vi "Buffered Continuous Packets.vi"(0 "Input Buffer":string, 3 "Packet definitions":T2(array[cluster])=[{"Cmd/SOP Byte"="ª", "Header Size"=6, "Len"=5, "Chksum Start"=1, "Chksum End"=-4, "InHdr"=TRUE}, {"Cmd/SOP Byte"="Â", "Header Size"=1, "Len"=31, "Chksum Start"=0, "Chksum End"=-2, "InHdr"=FALSE}]) -> (4 "Number of Remainder Bytes":i32, 6 "Number of Valid Records Found":i32, 7 "Remainder String":string, 9 "Valid Records Found":string[](array[string]), 10 "# of Bytes Rejected":i32)   [LabVIEW 2017]
panel:
  out "SOP":bool=TRUE
  in  "Current Pkt Definition":T1
  out "length":i32
  # "This VI pulls packets from the incoming data stream and outputs them in an array.  The only packets recognized are those that match one of the entries in the packet definitions array.   The types of packets recognized are either the single byte Inertia-Link/GX2/GX3 style commands or ASPP wireless packets.  You can input a custom set of packets to recognize.  The default recognizes the ASPP wireless packet and the \"C2\" command.  To add a single byte packet, set \"InHdr\" false, enter the command byte and reply Len, set Header Size to 1; Chksum Start o 0; Chksum End to -2."
  # "OUTPUT DATA"
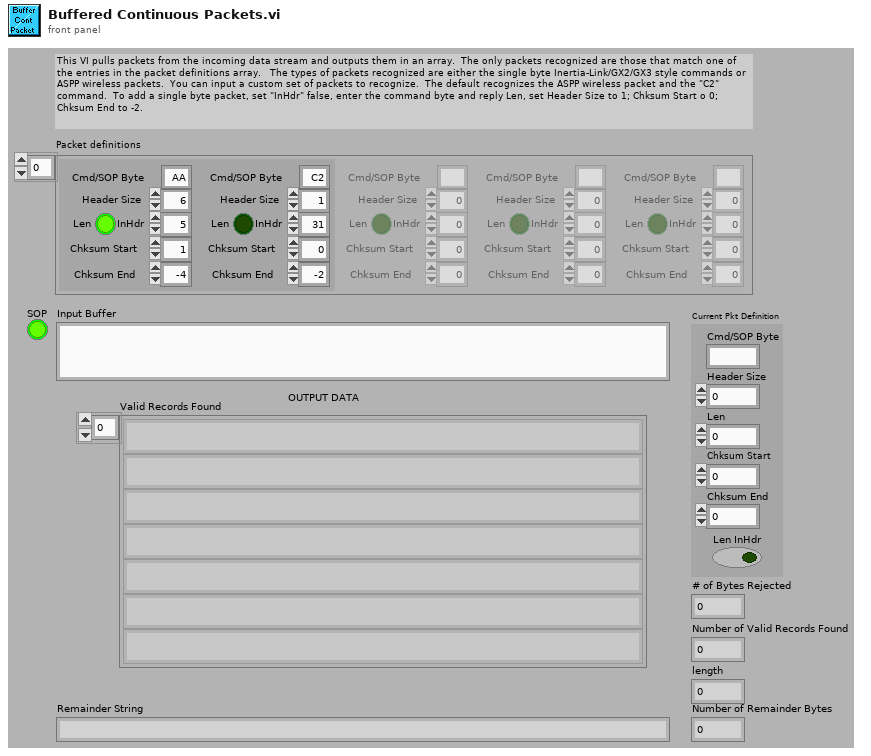
[diagram p1: front panel]
types:
  T1 = cluster{"Cmd/SOP Byte":string, "Header Size":u16, "Len":u16, "Chksum Start":u16, "Chksum End":i16, "Len InHdr":bool}
  T2 = cluster{"Cmd/SOP Byte":string, "Header Size":u16, "Len":u16, "Chksum Start":u16, "Chksum End":i16, "InHdr":bool}[]
  T3 = cluster{"Cmd/SOP Byte":string, "Header Size":u16, "Len":u16, "Chksum Start":u16, "Chksum End":i16, "IsLenB":bool}
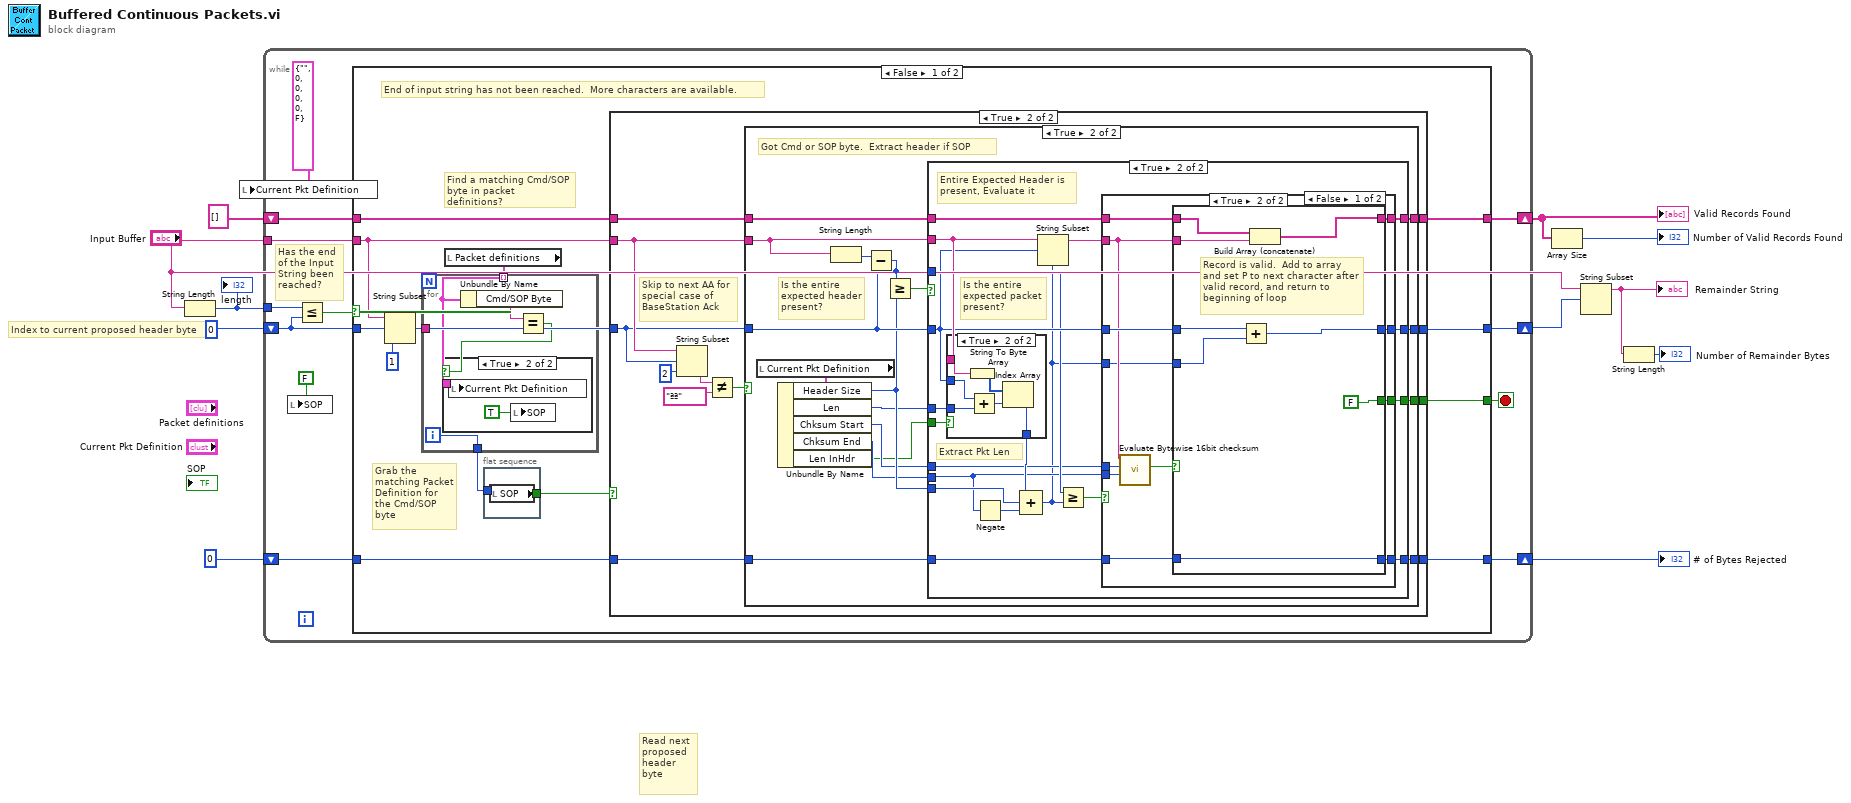
[diagram p0: block diagram]
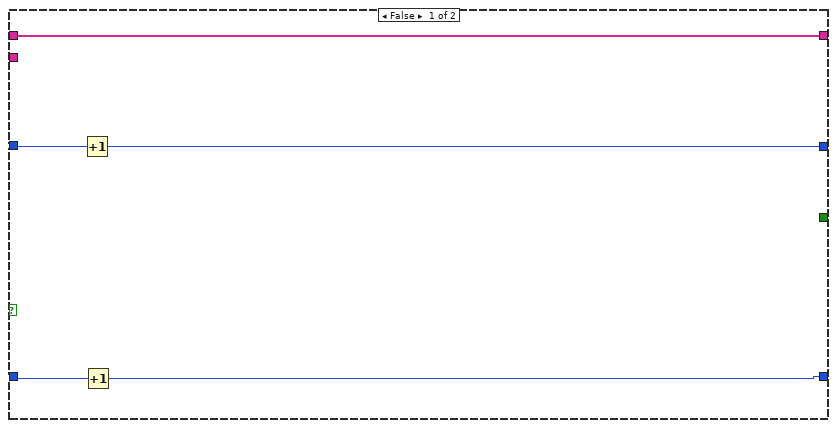
[diagram p3: hidden frame]
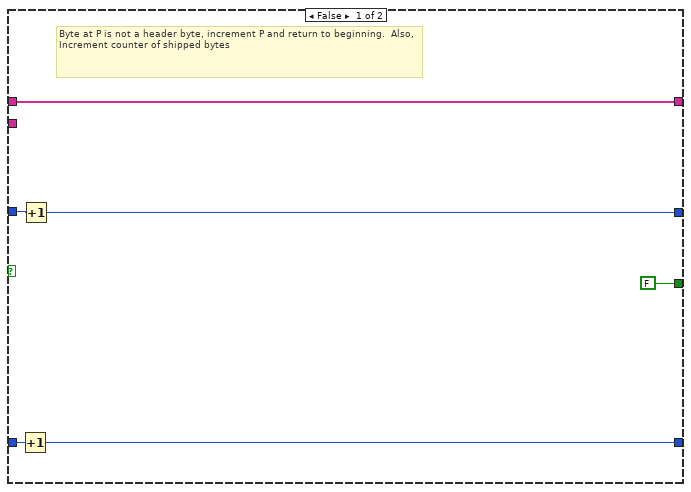
[diagram p4: hidden frame]
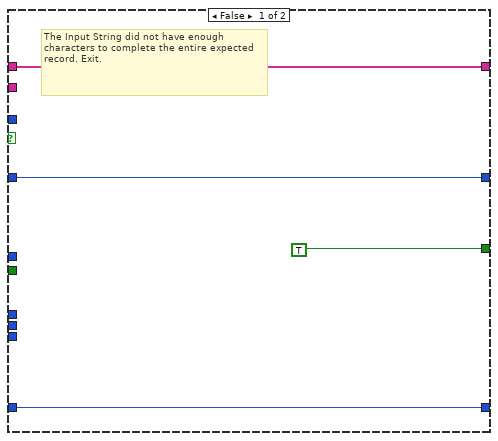
[diagram p5: hidden frame]
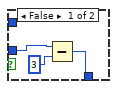
[diagram p6: hidden frame]
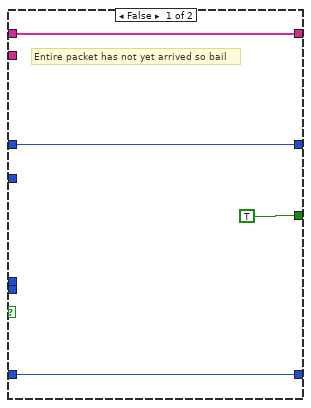
[diagram p7: hidden frame]
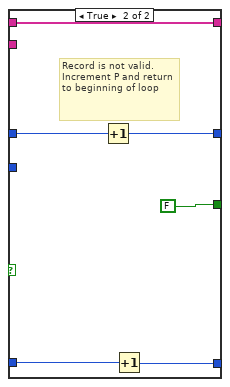
[diagram p8: hidden frame]
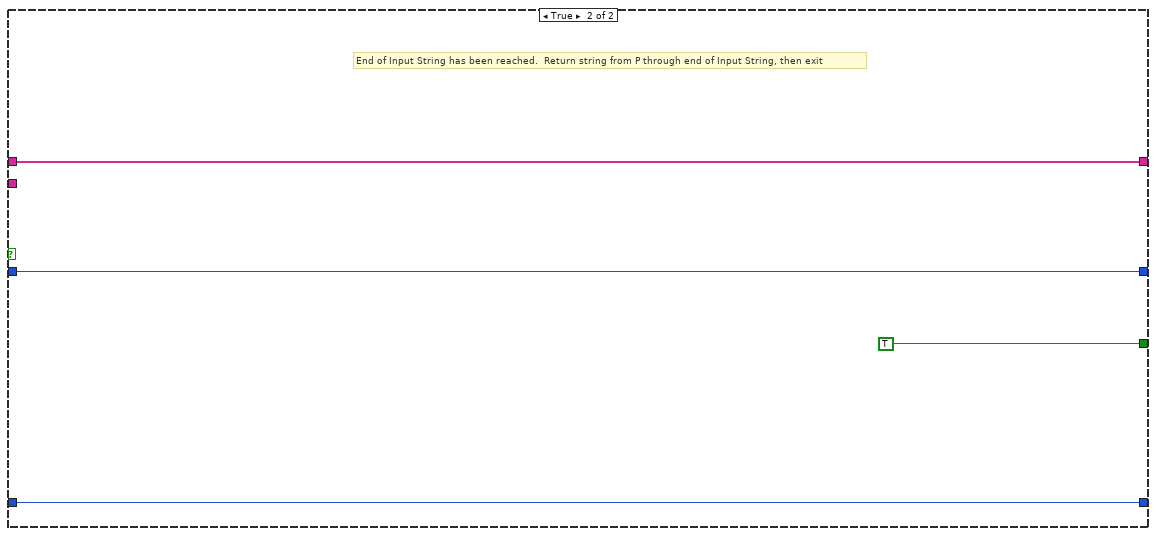
[diagram p9: hidden frame]
diagram:
  # "Read next proposed header byte"
  # "Index to current proposed header byte"
  n1 = String Length(string="Input Buffer") -> (length=w9:i32)
  "length" <- w9
  n2 = while {
    shift-right: [w16] -> w3
    shift-left: 0 -> [w21]
    tunnel: "Input Buffer" -> [w23]
    shift-right: [w18] -> w6
    shift-left: string[] [] -> [w19]
    tunnel: w9 -> [w22]
    shift-right: [w14] -> w7
    shift-left: 0 -> [w15]
    stop <- w17 stop-if-true
    # "Has the end of the Input String been reached?"
    n3 = local write "Current Pkt Definition"(T3 {"Cmd/SOP Byte"="", "Header Size"=0, "Len"=0, "Chksum Start"=0, "Chksum End"=0, "IsLenB"=FALSE} ("Cluster")) -> ()
    n4 = local write "SOP"(FALSE) -> ()
    n5 = Less Or Equal?(x=w22, y=w21) -> (x <= y?=w20:bool)
    n6 = case shown="False" w20 {
      tunnel: w23 -> [w33 _]
      tunnel: w21 -> [w32 w148]
      tunnel: w19 -> [w35 w150]
      tunnel: [w34 w150] -> w18
      tunnel: [w28 TRUE] -> w17
      tunnel: [w31 w148] -> w16
      tunnel: w15 -> [w30 w147]
      tunnel: [w29 w147] -> w14
      frame False {
        # "Grab the matching Packet Definition for the Cmd/SOP byte"
        # "Find a matching Cmd/SOP byte in packet definitions?"
        # "End of input string has not been reached.  More characters are available."
        n7 = String Subset(string=w33, offset (0)=w32, length (rest)=1 ("length (rest)")) -> (substring=w27:string)
        n8 = local read "Packet definitions"() -> (w24:T2)
        n9 = for {
          tunnel: w27 -> [w42]
          tunnel: [w39] -> w25
          tunnel: w24 -> [w38] mode=indexing
          i -> [w39]
          n10 = Unbundle By Name(w38) -> ("Cmd/SOP Byte"=w40:string)
          n11 = Equal?(x=w40, y=w42) -> (x = y?=w41:bool)
          n12 = case shown="True" w41 {
            tunnel: w38 -> [_ w44]
            frame False {
            }
            frame True {
              n13 = local write "Current Pkt Definition"(w44) -> ()
              n14 = local write "SOP"(TRUE) -> ()
            }
          }
        }
        n15 = flat-sequence {
          tunnel: [w37] -> w26
          tunnel: w25 -> [_]
          frame #0 {
            n16 = local read "SOP"() -> (w37:bool)
          }
        }
        n17 = case shown="True" w26 {
          tunnel: w35 -> [w49 w61]
          tunnel: [w49 w60] -> w34
          tunnel: w33 -> [_ w55]
          tunnel: w32 -> [w48 w54]
          tunnel: [w47 w59] -> w31
          tunnel: w30 -> [w46 w58]
          tunnel: [w45 w57] -> w29
          tunnel: [_ w56] -> w28
          frame False {
            n18 = Increment(x=w48) -> (x+1=w47:i32)
            n19 = Increment(x=w46) -> (x+1=w45:i32)
          }
          frame True {
            # "Skip to next AA for special case of BaseStation Ack"
            n20 = String Subset(string=w55, offset (0)=w54, length (rest)=2 ("length (rest)")) -> (substring=w51:string)
            n21 = Not Equal?(x=w51, y="ªª") -> (x != y?=w52:bool)
            n22 = case shown="True" w52 {
              tunnel: w61 -> [w67 w82]
              tunnel: [w67 w81] -> w60
              tunnel: w55 -> [_ w77]
              tunnel: w54 -> [w66 w75]
              tunnel: [w65 w83] -> w59
              tunnel: w58 -> [w64 w80]
              tunnel: [w63 w79] -> w57
              tunnel: [FALSE w78] -> w56
              frame False {
                # "Byte at P is not a header byte, increment P and return to beginning.  Also, Increment counter of shipped bytes"
                n23 = Increment(x=w64) -> (x+1=w63:i32)
                n24 = Increment(x=w66) -> (x+1=w65:i32)
              }
              frame True {
                # "Is the entire expected header present?"
                # "Got Cmd or SOP byte.  Extract header if SOP"
                n25 = local read "Current Pkt Definition"() -> (w73:T1)
                n26 = Unbundle By Name(w73) -> ("Header Size"=w72:u16, "Len"=w71:u16, "Chksum Start"=w70:u16, "Chksum End"=w69:i16, "Len InHdr"=w68:bool)
                n27 = String Length(string=w77) -> (length=w76:i32)
                n28 = Subtract(x=w76, y=w75) -> (x-y=w74:i32)
                n29 = Greater Or Equal?(x=w74, y=w72) -> (x >= y?=w84:bool)
                n30 = case shown="True" w84 {
                  tunnel: w77 -> [_ w100]
                  tunnel: w75 -> [w86 w95]
                  tunnel: [w86 w105] -> w83
                  tunnel: w82 -> [w88 w107]
                  tunnel: [w88 w106] -> w81
                  tunnel: w72 -> [_ w99]
                  tunnel: w80 -> [w87 w104]
                  tunnel: [w87 w103] -> w79
                  tunnel: [TRUE w90] -> w78
                  tunnel: w70 -> [_ w93]
                  tunnel: w69 -> [_ w92]
                  tunnel: w71 -> [_ w102]
                  tunnel: w74 -> [_ w94]
                  tunnel: w68 -> [_ w89]
                  frame False {
                    # "The Input String did not have enough characters to complete the entire expected record. Exit."
                  }
                  frame True {
                    # "Extract Pkt Len"
                    # "Is the entire expected packet present?"
                    # "Entire Expected Header is \npresent, Evaluate it"
                    n31 = case shown="True" w89 {
                      tunnel: w102 -> [w109 w111]
                      tunnel: w100 -> [_ w116]
                      tunnel: [w110 w113] -> w98
                      tunnel: w95 -> [_ w112]
                      frame False {
                        n32 = Subtract(x=w109, y=u16 3 ("x")) -> (x-y=w110:u16)
                      }
                      frame True {
                        n33 = String To Byte Array(string=w116) -> (unsigned byte array=w115:u8[])
                        n34 = Add(x=w112, y=w111) -> (x+y=w114:i32)
                        n35 = Index Array(array=w115, index=w114) -> (element=w113:u8)
                      }
                    }
                    n36 = Negate(x=w92) -> (-x=w97:i16)
                    n37 = Compound Arithmetic op=ADD(w98, w99, w97) -> (w91:u16)
                    n38 = String Subset(string=w100, offset (0)=w95, length (rest)=w91) -> (substring=w101:string)
                    n39 = Greater Or Equal?(x=w94, y=w91) -> (x >= y?=w96:bool)
                    n40 = case shown="True" w96 {
                      tunnel: w107 -> [w120 w127]
                      tunnel: [w120 w124] -> w106
                      tunnel: w101 -> [_ w128]
                      tunnel: w95 -> [w118 w131]
                      tunnel: [w118 w132] -> w105
                      tunnel: w104 -> [w119 w130]
                      tunnel: [w119 w129] -> w103
                      tunnel: w93 -> [_ w122]
                      tunnel: w92 -> [_ w121]
                      tunnel: w91 -> [_ w125]
                      tunnel: [TRUE w123] -> w90
                      frame False {
                        # "Entire packet has not yet arrived so bail"
                      }
                      frame True {
                        n41 = call "Evaluate Bytewise 16bit checksum.vi"("End Offset  for Checksum Calc"=w121, "Start Offset for Checksum Calc"=w122, "Intput String"=w128) -> ("Checksum Error"=w126:bool)  [unwired: 3 in, 3 out]
                        n42 = case shown="False" w126 {
                          tunnel: [w139 w146] -> w132
                          tunnel: w131 -> [w140 w145]
                          tunnel: w130 -> [w135 w144]
                          tunnel: [w135 w143] -> w129
                          tunnel: w128 -> [w138 _]
                          tunnel: w127 -> [w137 w142]
                          tunnel: w125 -> [w136 _]
                          tunnel: [w134 w142] -> w124
                          tunnel: [FALSE FALSE] -> w123
                          frame False {
                            # "Record is valid.  Add to array and set P to next character after valid record, and return to beginning of loop"
                            n43 = Add(x=w140, y=w136) -> (x+y=w139:i32)
                            n44 = Build Array (concatenate)(w137, w138) -> (w134:string[])
                          }
                          frame True {
                            # "Record is not valid.  Increment P and return to beginning of loop"
                            n45 = Increment(x=w145) -> (x+1=w146:i32)
                            n46 = Increment(x=w144) -> (x+1=w143:i32)
                          }
                        }
                      }
                    }
                  }
                }
              }
            }
          }
        }
      }
      frame True {
        # "End of Input String has been reached.  Return string from P through end of Input String, then exit"
      }
    }
  }
  "Valid Records Found" <- w6
  "# of Bytes Rejected" <- w7
  n47 = Array Size(array=w6) -> (size(s)=→"Number of Valid Records Found":i32)
  n48 = String Subset(string="Input Buffer", offset (0)=w3) -> (substring=w2:string)  [unwired: 1 in]
  "Remainder String" <- w2
  n49 = String Length(string=w2) -> (length=→"Number of Remainder Bytes":i32)
